vi "Main-Remote.vi"() -> ()   [LabVIEW 2019]
uses:
  Controller/F710PackedLibrary.lvlibp/stick.ctl
  <vilib>/myRIO/Instrument Drivers/Onboard IO/DIO/typedefs/DIO Reference.ctl
  <vilib>/myRIO/Common/Instrument Driver Framework/Utilities/typedefs/myRIO Generic Hardware Reference.ctl
  <vilib>/myRIO/Common/Instrument Driver Framework/Utilities/typedefs/Hardware Version Enum.ctl
  <vilib>/myRIO/Common/Instrument Driver Framework/Utilities/typedefs/myRIO v1.0 Reference.ctl
  <vilib>/myRIO/Common/Instrument Driver Framework/Utilities/typedefs/Generic FPGA Reference.ctl
  <vilib>/myRIO/Common/Instrument Driver Framework/myRIO v1.0/DIO/typedefs/DIO Channels List.ctl
  <vilib>/myRIO/Common/Instrument Driver Framework/myRIO v1.0/DIO/typedefs/DIO Channels Enum.ctl
  <vilib>/userDefined/High Color/nirio_resource_hc.ctl
  <vilib>/Platform/TimedLoop/XDataNode/timing_clust.ctl
  <vilib>/Platform/TimedLoop/XDataNode/nitl_modes.ctl
  <vilib>/Platform/TimedLoop/XDataNode/wakeup.ctl
  <vilib>/myRIO/Common/Instrument Driver Framework/Utilities/vis/Is FPGA Ref Available.vi
  <vilib>/myRIO/Common/Instrument Driver Framework/myRIO v1.0/DIO/vis/myRIO v1.1 Open DIO.vi
  <vilib>/myRIO/Instrument Drivers/Onboard IO/DIO/vis/Write.vi
  <vilib>/myRIO/Common/Instrument Driver Framework/Utilities/vis/Validate Channels.vi
  <vilib>/myRIO/Common/Instrument Driver Framework/myRIO v1.0/DIO/vis/myRIO v1.0 Reserve DIO.vi
  <vilib>/myRIO/Common/Instrument Driver Framework/myRIO v1.0/UART/vis/myRIO v1.0 Close UART.vi
  <vilib>/myRIO/Common/Instrument Driver Framework/myRIO v1.0/Resource Manager/vis/myRIO v1.0 Reserve Channel List.vi
  <vilib>/myRIO/Common/Instrument Driver Framework/myRIO v1.0/DIO/vis/myRIO v1.0 Build MUX Configuration DIO.vi
  <vilib>/myRIO/Common/Instrument Driver Framework/myRIO v1.0/Resource Manager/vis/myRIO v1.0 Reserve Channel.vi
  <vilib>/myRIO/Common/Instrument Driver Framework/myRIO v1.0/Resource Manager/vis/myRIO v1.0 Unreserve Channel.vi
  <vilib>/myRIO/Common/Instrument Driver Framework/myRIO v1.0/Resource Manager/vis/myRIO v1.0 Create Configuration List.vi
  <vilib>/myRIO/Common/Instrument Driver Framework/myRIO v1.0/Resource Manager/vis/myRIO v1.0 Build Mutex Name.vi
  <vilib>/Utility/VariantDataType/GetNumericInfo.vi
  <vilib>/Utility/error.llb/Error Cluster From Error Code.vi
  <vilib>/myRIO/Common/Instrument Driver Framework/myRIO v1.0/myRIO v1.1 Open.vi
  <vilib>/myRIO/Common/Instrument Driver Framework/Utilities/vis/IO Manager.vi
  <vilib>/myRIO/Common/Instrument Driver Framework/Utilities/vis/Configuration Manager.vi
  <vilib>/myRIO/Common/Instrument Driver Framework/myRIO v1.0/Resource Manager/vis/myRIO v1.0 Configure IO.vi
  <vilib>/myRIO/Common/Instrument Driver Framework/myRIO v1.0/myRIO v1.0 Close.vi
  <vilib>/myRIO/Common/Instrument Driver Framework/myRIO v1.0/DIO/vis/myRIO v1.0 Write DIO.vi
  <vilib>/myRIO/Common/Instrument Driver Framework/Utilities/vis/FPGA Ref Manager.vi
  <vilib>/myRIO/Common/Instrument Driver Framework/myRIO v1.0/myRIO v1.0 Reset FPGA.vi
  <vilib>/myRIO/Common/Instrument Driver Framework/myRIO v1.0/IRQ/vis/myRIO v1.0 IRQ Info FGV.vi
  <vilib>/myRIO/Common/Instrument Driver Framework/myRIO v1.0/IRQ/vis/myRIO v1.0 Timer IRQ Info FGV.vi
  <vilib>/myRIO/Common/Instrument Driver Framework/myRIO v1.0/IRQ/vis/myRIO v1.0 ISR Agent.vi
  <vilib>/myRIO/Instrument Drivers/Utilities/vis/Reset Index.vi
  <vilib>/myRIO/Common/Instrument Driver Framework/myRIO v1.0/Resource Manager/vis/myRIO v1.0 Block Write Resource Manager.vi
  <vilib>/myRIO/Express VI/Onboard Devices/LED/LED Express VI.xnode
  <vilib>/myRIO/Instrument Drivers/Onboard IO/DIO/vis/myRIO DIO Open.xnode
  <vilib>/platform/TimedLoop/XDataNode/XDataNode.xnode
  <vilib>/Platform/TimedLoop/XDataNode/XDNodeRunTimeDep.lvlib
  <vilib>/myRIO/Instrument Drivers/Utilities/Utilities.lvlib
  <vilib>/ptbypt/NI_PtbyPt.lvlib
  <vilib>/myRIO/Instrument Drivers/Onboard IO/DIO/DIO.lvlib
  Controller/F710PackedLibrary.lvlibp
panel:
  out "減速?":bool
  out "AI已上升?":bool
  out "中柱上升?":bool
  in  "伺服停止":bool
  in  "中柱停止":bool
  in  "AI停止":bool
  in  "移動停止":bool
  in  "停止讀值":bool
  in  "error in (no error)":errorcluster
  out "S-BUS Controller":T2 {"CH16" scale=-1024.0..1024.0; "CH15" scale=-1024.0..1024.0; "CH14" scale=-1024.0..1024.0; "CH13" scale=-1024.0..1024.0; "CH12" scale=-1024.0..1024.0; "CH11" scale=-1024.0..1024.0; "CH10" scale=-1024.0..1024.0; "CH9" scale=-1024.0..1024.0; "CH8" scale=-1024.0..1024.0; "CH7" scale=-1024.0..1024.0; "CH6" scale=-1024.0..1024.0; "CH5" scale=-1024.0..1024.0}
  out "error out":errorcluster
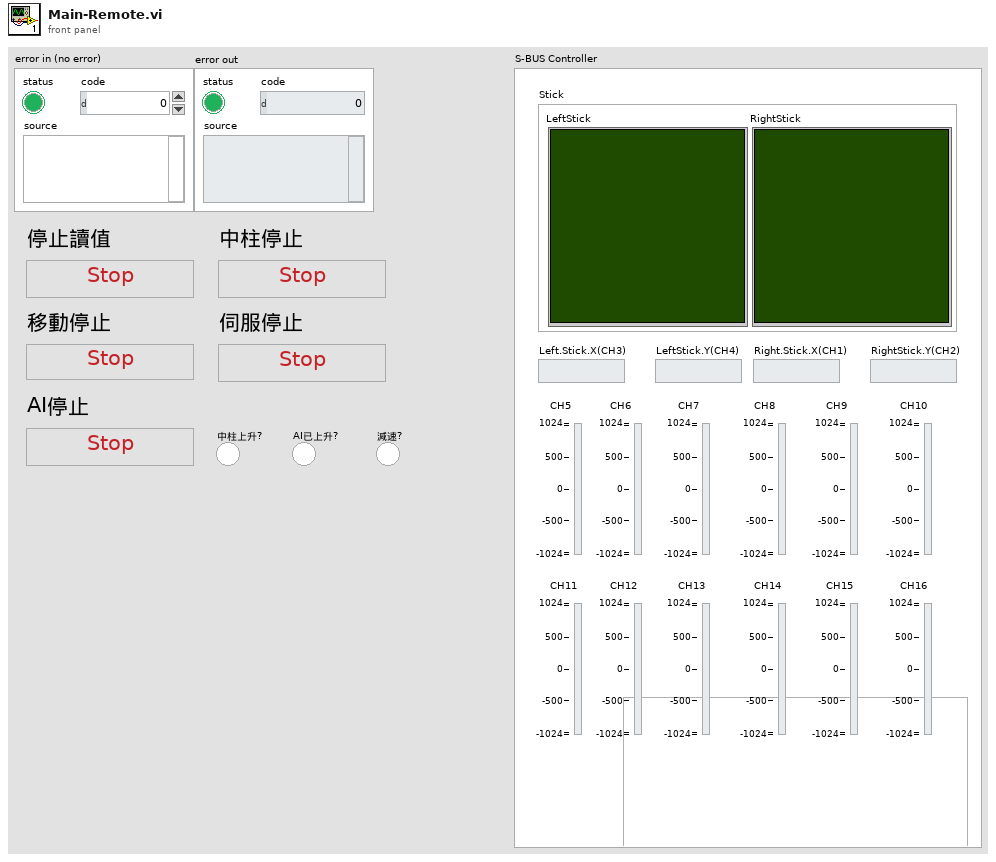
[diagram p1: front panel]
types:
  T1 = typedef "F710PackedLibrary.lvlibp/stick.ctl" = cluster{"X":dbl, "Y":dbl}[]
  T2 = cluster{"Stick":cluster{"LeftStick":T1, "RightStick":T1}, "Left.Stick.X(CH3)":dbl, "LeftStick.Y(CH4)":dbl, "Right.Stick.X(CH1)":dbl, "RightStick.Y(CH2)":dbl, "CH5":dbl, "CH6":dbl, "CH7":dbl, "CH8":dbl, "CH9":dbl, "CH10":dbl, "CH11":dbl, "CH12":dbl, "CH13":dbl, "CH14":dbl, "CH15":dbl, "CH16":dbl}
  T3 = typedef "I2C.lvlib/I2C Reference.ctl" = cluster{"myRIO Reference":T4, "I2C Channels Enum":T8, "I2C Configuration":T9}
  T4 = typedef "myRIO Generic Hardware Reference.ctl" = cluster{"myRIO Model":T5, "myRIO Hardware Reference":T6}
  T5 = typedef "Hardware Version Enum.ctl" = enum16{"Unknown", "myRIO-1900", "myRIO-1950", "roboRIO", "NI ELVIS RIO CM", "ELVIS III"}
  T6 = typedef "myRIO v1.0 Reference.ctl" = cluster{"Generic FPGA Reference":T7, "Allow multiple opens":bool}
  T7 = typedef "Generic FPGA Reference.ctl" = refnum<k20>
  T8 = typedef "I2C Channels Enum.ctl" = enum16{"Not Connected", "A/I2C", "B/I2C", "I2C/I2C"}
  T9 = typedef "I2C.lvlib/I2C Configuration.ctl" = cluster{"I2C Transfer Rate":T10}
  T10 = typedef "I2C.lvlib/I2C Transfer Rate.ctl" = enum16{"Standard mode (100 kbps)", "Fast mode (400 kbps)"}
  T11 = typedef "DIO.lvlib/DIO Reference.ctl" = cluster{"myRIO Reference":T4, "DIO Channels List":T12}
  T12 = typedef "DIO Channels List.ctl" = T13[]
  T13 = typedef "DIO Channels Enum.ctl" = enum16{"Not Connected", "C/DIO0", "C/DIO1", "C/DIO2", "C/DIO3", "C/DIO4", "C/DIO5", "C/DIO6", "C/DIO7", "A/DIO0", "A/DIO1", "A/DIO2", "A/DIO3", "A/DIO4", "A/DIO5", "A/DIO6", "A/DIO7", "A/DIO8", "A/DIO9", "A/DIO10", "A/DIO11", "A/DIO12", "A/DIO13", "A/DIO14", "A/DIO15", "A/DIO16", "A/DIO17", "A/DIO18", "A/DIO19", "B/DIO0", "B/DIO1", "B/DIO2", "B/DIO3", "B/DIO4", "B/DIO5", "B/DIO6", "B/DIO7", "B/DIO8", "B/DIO9", "B/DIO10", "B/DIO11", "B/DIO12", "B/DIO13", "B/DIO14", "B/DIO15", "B/DIO16", "B/DIO17", "B/DIO18", "B/DIO19", "LED0", "LED1", "LED2", "LED3", "Button0", "DIO/DIO0", "DIO/DIO1", "DIO/DIO2", "DIO/DIO3", "DIO/DIO4", "DIO/DIO5", "DIO/DIO6", "DIO/DIO7", "DIO/DIO8", "DIO/DIO9", "SPI/CS0", "SPI/CS1", "SPI/CS2", "SPI/CS3", "LED RADIO (Green)", "LED RADIO (Red)", "LED COMM (Green)", "LED COMM (Red)", "LED MODE (Green)", "LED MODE (Red)"}
  T14 = typedef "nirio_resource_hc.ctl" = tag
  T15 = cluster{"Stick":cluster{cluster{"X":bool, "Y":bool}[], cluster{"X":bool, "Y":bool}[]}, "Left.Stick.X(CH3)":bool, "LeftStick.Y(CH4)":bool, "Right.Stick.X(CH1)":bool, "RightStick.Y(CH2)":bool, "CH5":bool, "CH6":bool, "CH7":bool, "CH8":bool, "CH9":bool, "CH10":bool, "CH11":bool, "CH12":bool, "CH13":bool, "CH14":bool, "CH15":bool, "CH16":bool}
  T16 = typedef "XDNodeRunTimeDep.lvlib/timing_clust.ctl" = cluster{"Expected End [f-1]":u64, "Actual End [f-1]":u64, "Finished Late? [f-1]":bool, "Expected End [i-1]":u64, "Actual End [i-1]":u64, "Finished Late? [i-1]":bool, "Expected Start [i]":u64, "Actual Start [i]":u64, "Expected Start [f]":u64, "Actual Start [f]":u64, "Source Name":string, "Structure Name":string, "Period":i64, "Deadline":i64, "Offset":i64, "Start":i64, "Priority":i32, "Timeout":i32, "Mode":T17, "Wakeup Reason":T18, "Error":errorcluster, "Source Type":string, "Secondary Source Type":string, "Global End Time":u64, "Global Start Time":u64, "Frame Duration":u64, "Iteration Duration":u64, "Assigned CPU":i32, "I/O Scan Engine Mode":u32}
  T17 = typedef "XDNodeRunTimeDep.lvlib/nitl_modes.ctl" = enum32{"No Change", "Process missed periods, maintain original phase", "Discard missed periods, maintain original phase", "Process missed periods, ignore original phase", "Discard missed periods, ignore original phase"}
  T18 = typedef "XDNodeRunTimeDep.lvlib/wakeup.ctl" = enum32{"Normal", "Aborted", "Asynchronous wakeup", "Timing source error", "Timed loop error", "Timeout"}
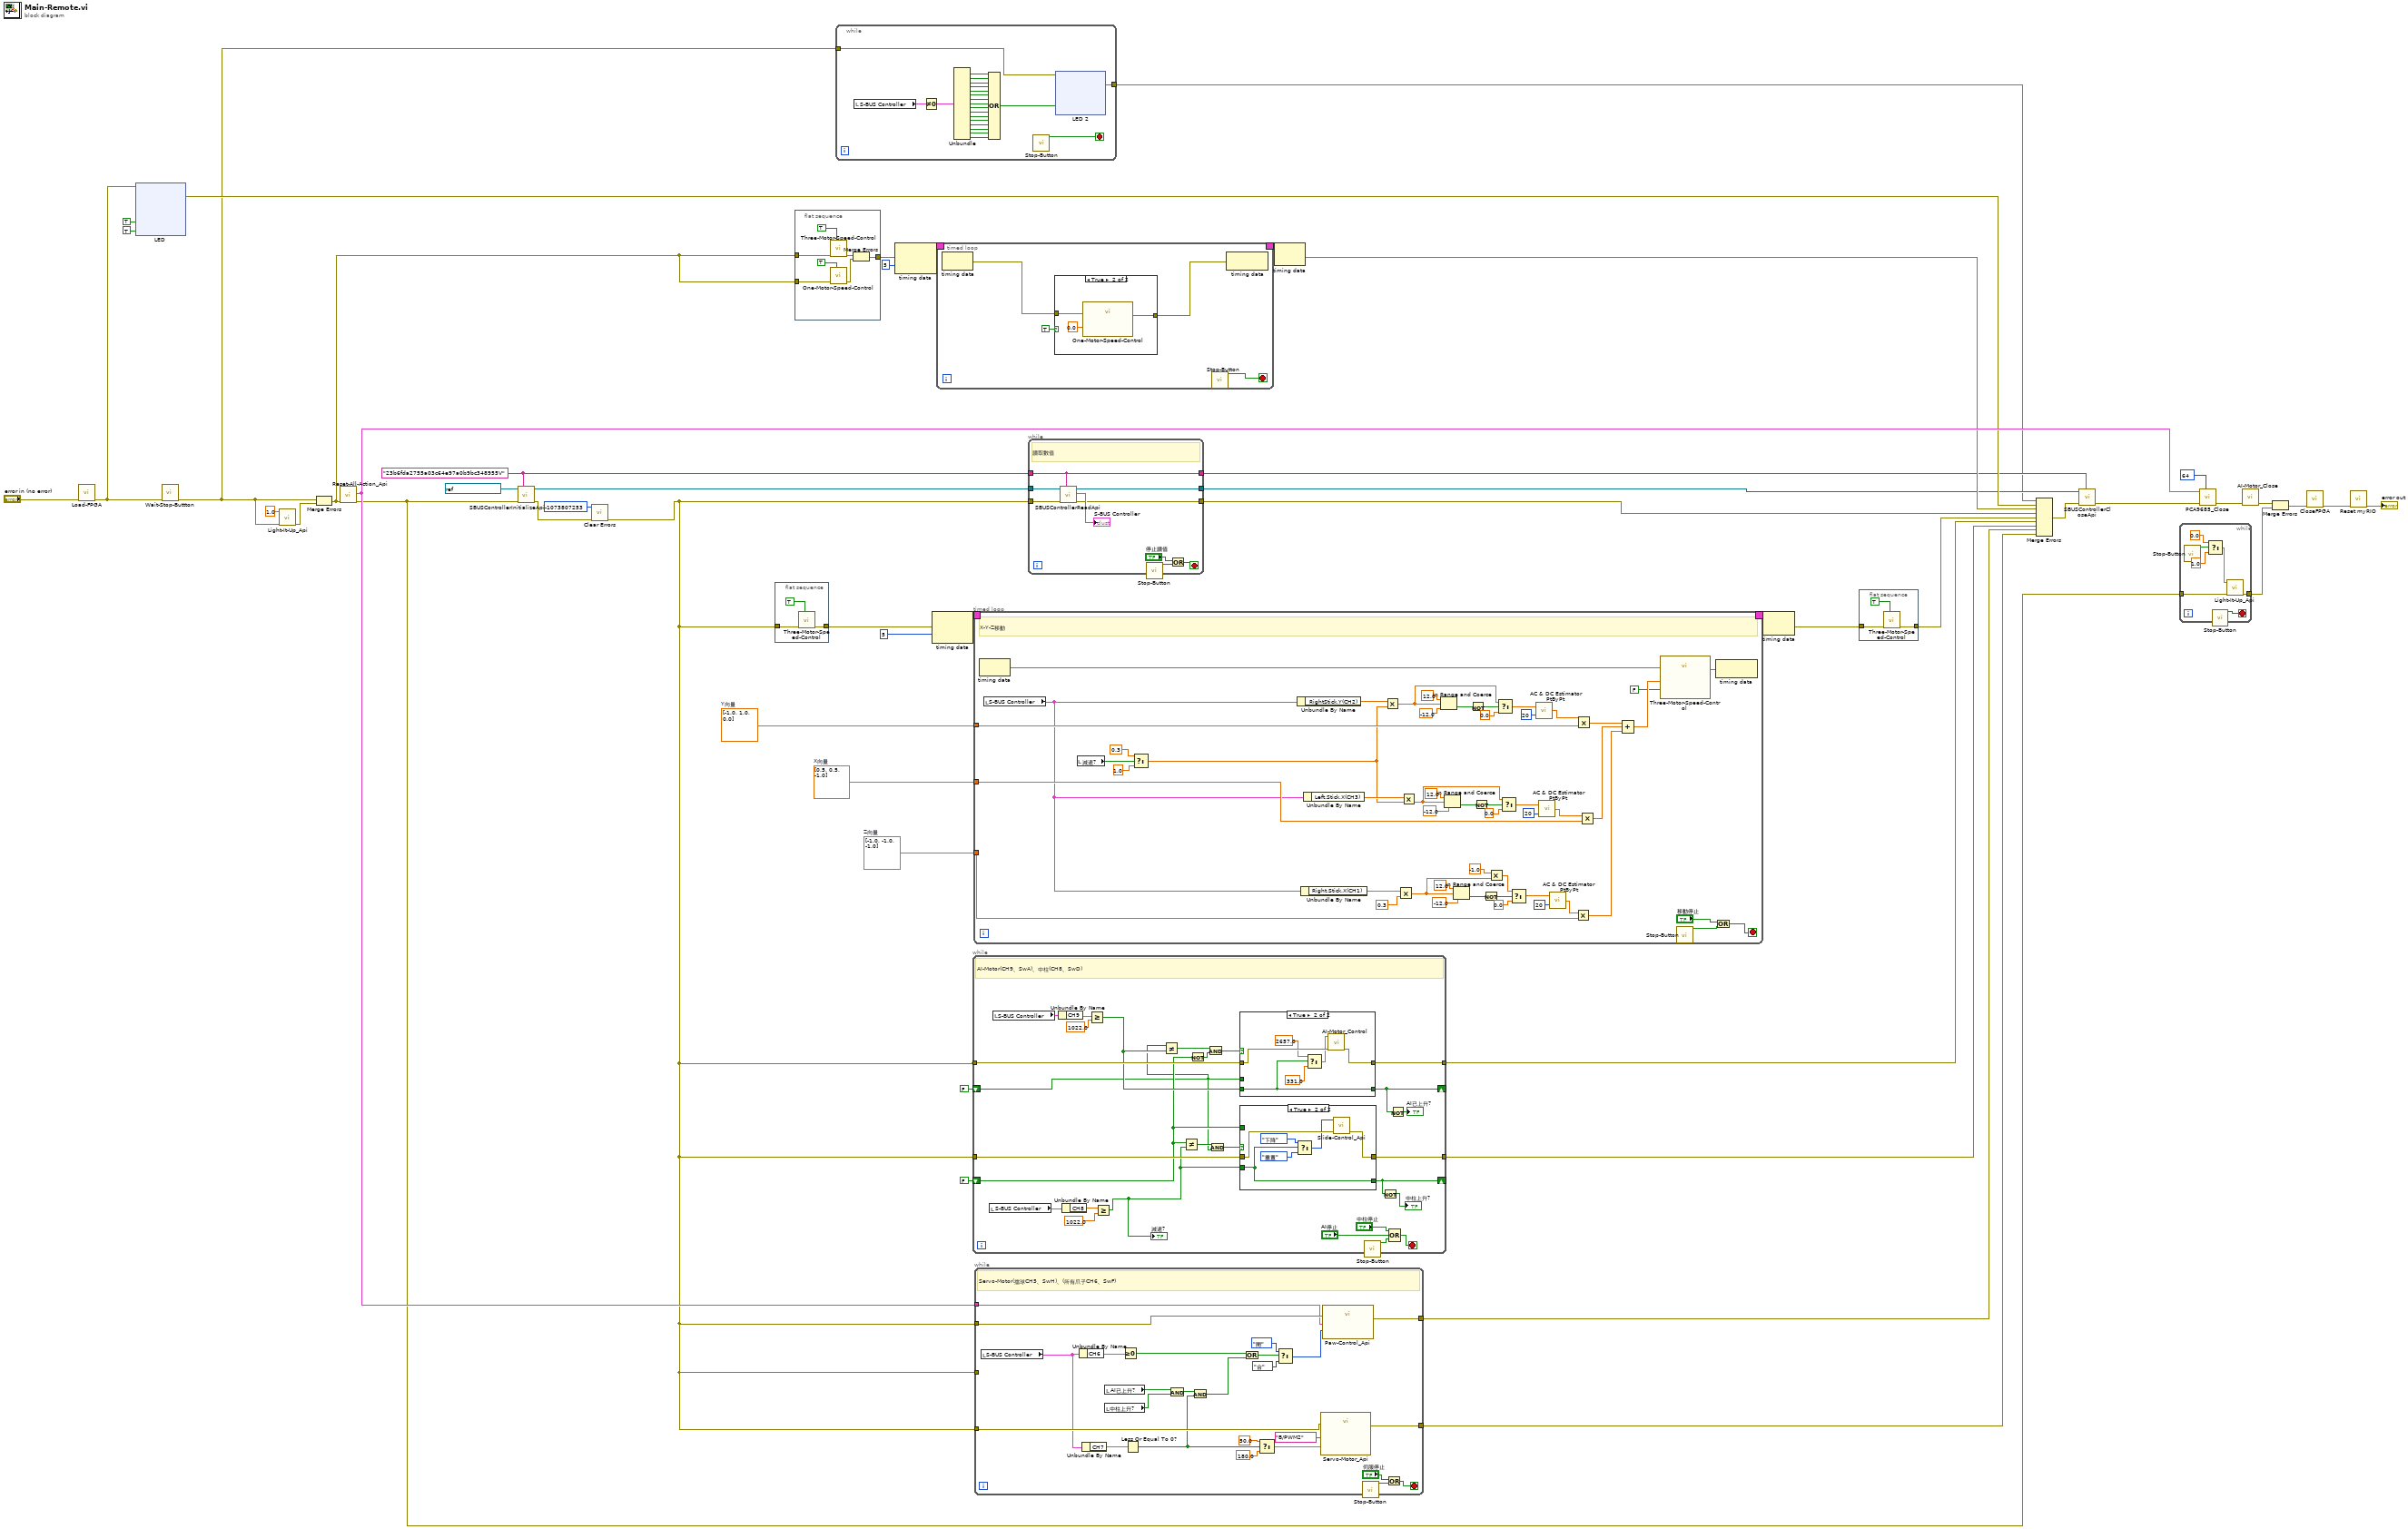
[diagram p0: block diagram]
diagram:
  w15 = "23b6fda2755a03c64e97a0b9bc348955V" ("設備授權碼")
  w42 = dbl[] [-1.0, -1.0, -1.0]  # Z向量
  w43 = dbl[] [0.5, 0.5, -1.0]  # X向量
  w40 = dbl[] [-1.0, 1.0, 0.0]  # Y向量
  n1 = call "Load-FPGA.vi"("Error In"="error in (no error)") -> ("Error Out"=w5:errorcluster)  [unwired: 10 in]
  n2 = xnode "LED"("LED0"=TRUE, "LED1"=TRUE, "error in (no error)"=w5) -> ("error out"=w20:errorcluster)
  n3 = call "Wait-Stop-Buttton.vi"("Error In"=w5) -> ("Error Out"=w3:errorcluster)  [unwired: 10 in]
  n4 = call "Light-It-Up_Api.vi"("error in (no error)"=w3, "Duty Cycle"=1.0) -> ("error out"=w23:errorcluster)  [unwired: 9 in]
  n5 = Merge Errors(w3, w23) -> (w6:errorcluster)
  n6 = call "Reset-All-Action_Api.vi"("Error In"=w6) -> ("Error Out"=w18:errorcluster, "I2C Ref Out"=w35:T3)  [unwired: 8 in, 1 out]
  n7 = call "SBUSControllerInitializeApi.vi"("設備授權碼"=w15, "error in (no error)"=w18, "VISA Refnum in"=refnum<visa-resource-name> "ASRL2::INSTR") -> ("error out"=w8:errorcluster, "VISA Refnum out"=w17:refnum<visa-resource-name>)  [unwired: 7 in]
  n8 = call <vilib>:"Clear Errors.vi"("error in (no error)"=w8, "specific error code to clear (0: all)"=-1073807253) -> ("error out"=w1:errorcluster)  [unwired: 4 in, 1 out]
  n9 = flat-sequence {
    tunnel: w1 -> [w52]
    tunnel: [w51] -> w47
    frame #0 {
      n10 = call "Three-Motor-Speed-Control.vi"("Reset"=TRUE, "Error In"=w52) -> ("Error Out"=w51:errorcluster)  [unwired: 9 in]
    }
  }
  n11 = flat-sequence {
    tunnel: w6 -> [w60]
    tunnel: w6 -> [w59]
    tunnel: [w56] -> w29
    frame #0 {
      n12 = call "Three-Motor-Speed-Control.vi"("Reset"=TRUE, "Error In"=w60) -> ("Error Out"=w58:errorcluster)  [unwired: 9 in]
      n13 = call "One-Motor-Speed-Control.vi"("Reset"=TRUE, "Error In"=w59) -> ("Error Out"=w57:errorcluster)  [unwired: 9 in]
      n14 = Merge Errors(w58, w57) -> (w56:errorcluster)
    }
  }
  n15 = while {
    tunnel: w3 -> [w63]
    tunnel: [w62] -> w4
    stop <- w61 stop-if-true
    n16 = local read "S-BUS Controller"() -> (w82:T2)
    n17 = Not Equal To 0?(x=w82) -> (x != 0?=w81:T15)
    n18 = Unbundle(w81) -> ("Left.Stick.X(CH3)"=w65:bool, "LeftStick.Y(CH4)"=w66:bool, "Right.Stick.X(CH1)"=w67:bool, "RightStick.Y(CH2)"=w68:bool, "CH5"=w69:bool, "CH6"=w70:bool, "CH7"=w71:bool, "CH8"=w72:bool, "CH9"=w73:bool, "CH10"=w74:bool, "CH11"=w75:bool, "CH12"=w76:bool, "CH13"=w77:bool, "CH14"=w78:bool, "CH15"=w79:bool, "CH16"=w80:bool)  [unwired: 1 out]
    n19 = Compound Arithmetic op=OR(w65, w66, w67, w68, w69, w70, w71, w72, w73, w74, w75, w76, w77, w78, w79, w80) -> (w64:bool)
    n20 = call "Stop-Button.vi"() -> ("顯示按下?"=w61:bool)  [unwired: 10 in, 1 out]
    n21 = xnode "LED 2"("LED3"=w64, "error in (no error)"=w63) -> ("error out"=w62:errorcluster)
  }
  n22 = node-c288(w29, i64 5 ("Period")) -> (w32:T16)
  n23 = node-c288(w47, i64 5 ("Period")) -> (w46:T16)
  n24 = timed-loop {
    timing: w32 -> [_]
    timing-out: [_] -> w31
    stop <- w121 stop-if-true
    n25 = node-c288() -> (w120:errorcluster)  [unwired: 1 in]
    n26 = case shown="True" TRUE {
      tunnel: w120 -> [w122 w124]
      tunnel: [w122 w123] -> w119
      frame False {
      }
      frame True {
        n27 = call "One-Motor-Speed-Control.vi"("Error In"=w124, "速度(秒/度)"=0.0) -> ("Error Out"=w123:errorcluster)  [unwired: 9 in]
      }
    }
    n28 = call "Stop-Button.vi"() -> ("顯示按下?"=w121:bool)  [unwired: 10 in, 1 out]
    n29 = node-c288(w119) -> ()  [unwired: 1 out]
  }
  n30 = while {
    tunnel: [w147] -> w37
    tunnel: [w145] -> w36
    tunnel: w1 -> [w146]
    tunnel: w1 -> [w144]
    shift-right: [w134] -> _
    shift-left: FALSE -> [w136]
    shift-right: [w131] -> _
    shift-left: FALSE -> [w135]
    stop <- w156 stop-if-true
    # "AI-Motor(CH9、SwA)、中柱(CH8、SwD)"
    n31 = local read "S-BUS Controller"() -> (w149:T2)
    n32 = local read "S-BUS Controller"() -> (w154:T2)
    n33 = Unbundle By Name(w154) -> ("CH9"=w152:dbl)
    n34 = Unbundle By Name(w149) -> ("CH8"=w150:dbl)
    n35 = Greater Or Equal?(x=w152, y=1022.0) -> (x >= y?=w142:bool)
    n36 = Greater Or Equal?(x=w150, y=1022.0) -> (x >= y?=w143:bool)
    "減速?" <- w143
    n37 = Not Equal?(x=w135, y=w142) -> (x != y?=w139:bool)
    n38 = Not Equal?(x=w136, y=w143) -> (x != y?=w141:bool)
    n39 = Not(x=w136) -> (.not. x?=w137:bool)
    n40 = And(x=w139, y=w137) -> (x .and. y?=w138:bool)
    n41 = And(x=w141, y=w135) -> (x .and. y?=w140:bool)
    n42 = case shown="True" w138 {
      tunnel: [w167 w172] -> w147
      tunnel: w146 -> [w167 w173]
      tunnel: [w166 w168] -> w131
      tunnel: w142 -> [_ w168]
      tunnel: w135 -> [w166 _]
      frame False {
      }
      frame True {
        n43 = Select(t=2657.0, s=w168, f=331.0) -> (s? t:f=w171:dbl)
        n44 = call "AI-Motor_Control.vi"("Error In"=w173, "目標位置(0~4095)"=w171) -> ("Error Out"=w172:errorcluster)  [unwired: 9 in]
      }
    }
    n45 = case shown="True" w140 {
      tunnel: [w159 w163] -> w145
      tunnel: w144 -> [w159 w164]
      tunnel: [w158 w165] -> w134
      tunnel: w143 -> [_ w165]
      tunnel: w136 -> [w158 _]
      frame False {
      }
      frame True {
        n46 = Select(t=enum16{"重置", "下降"}."下降" ("狀態選擇"), s=w165, f=enum16{"重置", "下降"}."重置" ("狀態選擇")) -> (s? t:f=w160:enum16{"重置", "下降"})
        n47 = call "Slide-Control_Api.vi"("Error In"=w164, "狀態選擇"=w160) -> ("Error Out"=w163:errorcluster)  [unwired: 9 in]
      }
    }
    n48 = call "Stop-Button.vi"() -> ("顯示按下?"=w157:bool)  [unwired: 10 in, 1 out]
    n49 = Not(x=w134) -> (.not. x?=→"中柱上升?":bool)
    n50 = Compound Arithmetic op=OR("中柱停止", "AI停止", w157) -> (w156:bool)
    n51 = Not(x=w131) -> (.not. x?=→"AI已上升?":bool)
  }
  n52 = timed-loop {
    timing: w46 -> [_]
    timing-out: [_] -> w45
    tunnel: w40 -> [w183]
    tunnel: w43 -> [w207]
    tunnel: w42 -> [w200]
    stop <- w179 stop-if-true
    # "X-Y-Z移動"
    n53 = node-c288() -> (w223:errorcluster)  [unwired: 1 in]
    n54 = local read "S-BUS Controller"() -> (w182:T2)
    n55 = local read "減速?"() -> (w178:bool)
    n56 = Select(t=0.3, s=w178, f=1.0) -> (s? t:f=w175:dbl)
    n57 = Unbundle By Name(w182) -> ("RightStick.Y(CH2)"=w217:dbl)
    n58 = Unbundle By Name(w182) -> ("Right.Stick.X(CH1)"=w187:dbl)
    n59 = Unbundle By Name(w182) -> ("Left.Stick.X(CH3)"=w208:dbl)
    n60 = Multiply(x=w217, y=w175) -> (x*y=w186:dbl)
    n61 = Multiply(x=w187, y=0.3) -> (x*y=w189:dbl)
    n62 = Multiply(x=w208, y=w175) -> (x*y=w185:dbl)
    n63 = In Range and Coerce(upper limit=12.0, x=w186, lower limit=-12.0) -> (In Range?=w220:bool)  [unwired: 1 out]
    n64 = In Range and Coerce(upper limit=12.0, x=w185, lower limit=-12.0) -> (In Range?=w214:bool)  [unwired: 1 out]
    n65 = In Range and Coerce(upper limit=12.0, x=w189, lower limit=-12.0) -> (In Range?=w204:bool)  [unwired: 1 out]
    n66 = Not(x=w220) -> (.not. x?=w219:bool)
    n67 = Not(x=w214) -> (.not. x?=w215:bool)
    n68 = Not(x=w204) -> (.not. x?=w203:bool)
    n69 = Multiply(x=-1.0, y=w189) -> (x*y=w188:dbl)
    n70 = Select(t=w186, s=w219, f=0.0) -> (s? t:f=w199:dbl)
    n71 = Select(t=w185, s=w215, f=0.0) -> (s? t:f=w194:dbl)
    n72 = Select(t=w188, s=w203, f=0.0) -> (s? t:f=w195:dbl)
    n73 = call <vilib>:"AC & DC Estimator PtByPt.vi"("signal"=w199, "sample length"=20) -> ("DC estimate (V)"=w192:dbl)  [unwired: 1 in, 2 out]
    n74 = call <vilib>:"AC & DC Estimator PtByPt.vi"("signal"=w194, "sample length"=20) -> ("DC estimate (V)"=w193:dbl)  [unwired: 1 in, 2 out]
    n75 = call <vilib>:"AC & DC Estimator PtByPt.vi"("signal"=w195, "sample length"=20) -> ("DC estimate (V)"=w191:dbl)  [unwired: 1 in, 2 out]
    n76 = Multiply(x=w191, y=w200) -> (x*y=w201:dbl[])
    n77 = Multiply(x=w192, y=w183) -> (x*y=w211:dbl[])
    n78 = Multiply(x=w193, y=w207) -> (x*y=w210:dbl[])
    n79 = Compound Arithmetic op=ADD(w211, w210, w201) -> (w209:dbl[])
    n80 = call "Three-Motor-Speed-Control.vi"("Reset"=FALSE, "Error In"=w223, "速度(秒/度)"=w209) -> ("Error Out"=w224:errorcluster)  [unwired: 8 in]
    n81 = call "Stop-Button.vi"() -> ("顯示按下?"=w180:bool)  [unwired: 10 in, 1 out]
    n82 = Or(x="移動停止", y=w180) -> (x .or. y?=w179:bool)
    n83 = node-c288(w224) -> ()  [unwired: 1 out]
  }
  n84 = while {
    tunnel: w1 -> [w245]
    tunnel: w1 -> [_]
    tunnel: w1 -> [w248]
    tunnel: [w247] -> w34
    tunnel: w35 -> [w230]
    tunnel: [w244] -> w33
    stop <- w252 stop-if-true
    # "Servo-Motor(擋球CH5、SwH)、(所有爪子CH6、SwF)"
    n85 = local read "S-BUS Controller"() -> (w246:T2)
    n86 = Unbundle By Name(w246) -> ("CH6"=w235:dbl)
    n87 = Unbundle By Name(w246) -> ("CH7"=w234:dbl)
    n88 = local read "中柱上升?"() -> (w237:bool)
    n89 = local read "AI已上升?"() -> (w238:bool)
    n90 = Greater Or Equal To 0?(x=w235) -> (x >= 0?=w240:bool)
    n91 = Less Or Equal To 0?(x=w234) -> (x <= 0?=w233:bool)
    n92 = And(x=w238, y=w237) -> (x .and. y?=w236:bool)
    n93 = And(x=w236, y=w233) -> (x .and. y?=w232:bool)
    n94 = Or(x=w240, y=w232) -> (x .or. y?=w239:bool)
    n95 = Select(t=50.0, s=w233, f=180.0) -> (s? t:f=w231:dbl)
    n96 = Select(t=enum16{"開", "合"}."開", s=w239, f=enum16{"開", "合"}."合") -> (s? t:f=w241:enum16{"開", "合"})
    n97 = call "Servo-Motor_Api.vi"("角度"=w231, "Error In"=w248, "伺服馬達角位"=tag "B/PWM2") -> ("Error Out"=w247:errorcluster)  [unwired: 8 in]
    n98 = call "Paw-Control_Api.vi"("I2C Ref In"=w230, "Error In"=w245, "夾爪動作"=w241) -> ("error out"=w244:errorcluster)  [unwired: 8 in]
    n99 = call "Stop-Button.vi"() -> ("顯示按下?"=w254:bool)  [unwired: 10 in, 1 out]
    n100 = Or(x="伺服停止", y=w254) -> (x .or. y?=w252:bool)
  }
  n101 = while {
    tunnel: w17 -> [w259]
    tunnel: w1 -> [w257]
    tunnel: [w260] -> w12
    tunnel: [w255] -> w44
    tunnel: w15 -> [w258]
    tunnel: [w258] -> w11
    stop <- w263 stop-if-true
    # "讀取數值"
    n102 = call "SBUSControllerReadApi.vi"("設備授權碼"=w258, "error in (no error)"=w257, "VISA Refnum in"=w259) -> ("error out"=w255:errorcluster, "S-BUS Controller"=→"S-BUS Controller":T2, "VISA Refnum out"=w260:refnum<visa-resource-name>)  [unwired: 6 in]
    n103 = call "Stop-Button.vi"() -> ("顯示按下?"=w262:bool)  [unwired: 10 in, 1 out]
    n104 = Or(x="停止讀值", y=w262) -> (x .or. y?=w263:bool)
  }
  n105 = node-c288(w31) -> (w19:errorcluster)
  n106 = node-c288(w45) -> (w49:errorcluster)
  n107 = flat-sequence {
    tunnel: w49 -> [w265]
    tunnel: [w264] -> w48
    frame #0 {
      n108 = call "Three-Motor-Speed-Control.vi"("Reset"=TRUE, "Error In"=w265) -> ("Error Out"=w264:errorcluster)  [unwired: 9 in]
    }
  }
  n109 = Merge Errors(w4, w20, w19, w44, w48, w37, w36, w33, w34) -> (w13:errorcluster)
  n110 = call "SBUSControllerCloseApi.vi"("設備授權碼"=w11, "error in (no error)"=w13, "VISA Refnum in"=w12) -> ("error out"=w14:errorcluster)  [unwired: 8 in]
  n111 = while {
    tunnel: w18 -> [w268]
    tunnel: [w273] -> w25
    stop <- w267 stop-if-true
    n112 = call "Stop-Button.vi"() -> ("顯示按下?"=w271:bool)  [unwired: 10 in, 1 out]
    n113 = Select(t=0.0, s=w271, f=1.0) -> (s? t:f=w272:dbl)
    n114 = call "Stop-Button.vi"() -> ("顯示按下?"=w267:bool)  [unwired: 10 in, 1 out]
    n115 = call "Light-It-Up_Api.vi"("error in (no error)"=w268, "Duty Cycle"=w272) -> ("error out"=w273:errorcluster)  [unwired: 9 in]
  }
  n116 = call "PCA9685_Close.vi"("驅動板位址(0x40)"=u8 64, "Error In"=w14, "I2C Ref In"=w35) -> ("Error Out"=w28:errorcluster)  [unwired: 8 in]
  n117 = call "AI-Motor_Close.vi"("Error In"=w28) -> ("Error Out"=w26:errorcluster)  [unwired: 10 in]
  n118 = Merge Errors(w26, w25) -> (w27:errorcluster)
  n119 = call "CloseFPGA.vi"("Error In"=w27) -> ("Error Out"=w38:errorcluster)  [unwired: 10 in]
  n120 = call <vilib>:"Reset myRIO.vi"("error in (no error)"=w38) -> ("error out"=→"error out":errorcluster)  [unwired: 10 in]
